vi "Pre Launch Init.vi"(11 "LTI ULS Actor in":refnum<class "LTI ULS Actor.lvclass">) -> (0 "error out":errorcluster, 3 "LTI ULS Actor out":refnum<class "LTI ULS Actor.lvclass">)   [LabVIEW 2018, in "LTI ULS Actor.lvlib" / "LTI ULS Actor.lvclass"]
doc: "Sends a high priority message to it's self to notify the monitor that it's spawned. If it's in the runtime environment, this message is never sent, meaning the monitor will never spawn\n\nCopyright: MGI\nAuthored by: Derek Trepanier"
uses:
  LTI ULS Actor.lvclass
  LTI ULS Actor.lvclass/LTI ULS Actor.ctl
  Sensor Actor/Sensor/Sensor.lvclass
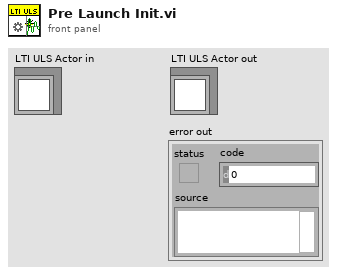
[diagram p1: front panel]
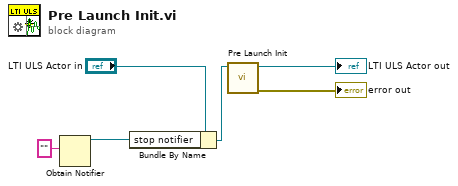
[diagram p0: block diagram]
diagram:
  n1 = Obtain Notifier(notification data type="") -> (notifier out=w1:refnum<notifier>)  [unwired: 3 in, 2 out]
  n2 = Bundle By Name(cluster="LTI ULS Actor in", "stop notifier"=w1) -> (w3:refnum<class "LTI ULS Actor.lvclass">)
  n3 = call-parent "Pre Launch Init.vi"("Sensor in"=w3) -> ("error out"=→"error out":errorcluster, "Sensor out"=→"LTI ULS Actor out":refnum<class "LTI ULS Actor.lvclass">)  [unwired: 9 in]
